vi "Untitled 4 (SubVI).vi"(6 "4":dbl, 9 "3":dbl, 10 "2":dbl, 11 "1":dbl) -> (1 "X Left":dbl, 2 "Y Left":dbl, 3 "Sum Left":dbl)   [LabVIEW 2019]
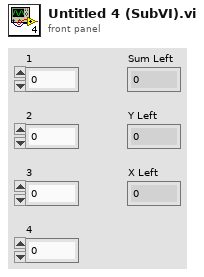
[diagram p1: front panel]
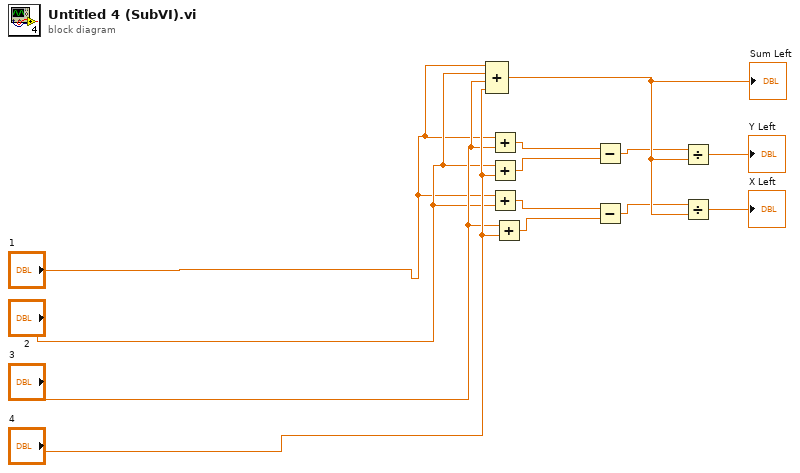
[diagram p0: block diagram]
diagram:
  n1 = Compound Arithmetic op=ADD("1", "2", "3", "4") -> (w11:dbl)
  "Sum Left" <- w11
  n2 = Add(x="1", y="3") -> (x+y=w1:dbl)
  n3 = Add(x="2", y="4") -> (x+y=w2:dbl)
  n4 = Add(x="1", y="2") -> (x+y=w3:dbl)
  n5 = Add(x="3", y="4") -> (x+y=w4:dbl)
  n6 = Subtract(x=w1, y=w2) -> (x-y=w10:dbl)
  n7 = Subtract(x=w3, y=w4) -> (x-y=w9:dbl)
  n8 = Divide(x=w10, y=w11) -> (x/y=→"Y Left":dbl)
  n9 = Divide(x=w9, y=w11) -> (x/y=→"X Left":dbl)
